vi "TDK正向工况电流-继电器控制 - 副本.vi"() -> ()   [LabVIEW 2020]
uses:
  <vilib>/Utility/file.llb/Read Delimited Spreadsheet (DBL).vi
  <instrlib>/TDK-Lambda G Series/TDK-Lambda G Series.lvlib
panel:
  out "耐久2":dbl[][](array[numeric])
  out "快充2":dbl[][](array[numeric])
  in  "耐久2":path
  in  "快充2":path
  in  "耐久循环次数2":i32
  in  "快充循环次数2":i32
  out "完成耐久循环 2":i32
  out "完成快充循环 2":i32
  in  "精度":i16
  out "?":bool
  in  "电源台数":dbl=3.0
  in  "TDK地址":refnum<visa-resource-name>="COM15"
  in  "耐久循环次数":i32
  in  "file path (dialog if empty) 2":path caption="耐久工况"
  out "耐久工况":string[][](table)
  out "快充工况":string[][](table)
  in  "file path (dialog if empty)":path caption="快充工况"
  out "已成大循环数":i32
  out "完成耐久循环":i32
  out "完成快充循环":i32
  in  "工况切换地址":refnum<visa-resource-name>
  in  "停止":bool
  in  "快充循环次数":i32
  in  "大循环次数":i32
  in  "耐久工况":cluster{"CH1":bool, "CH2":bool}
  in  "快充工况":cluster{"CH1":bool, "CH2":bool}
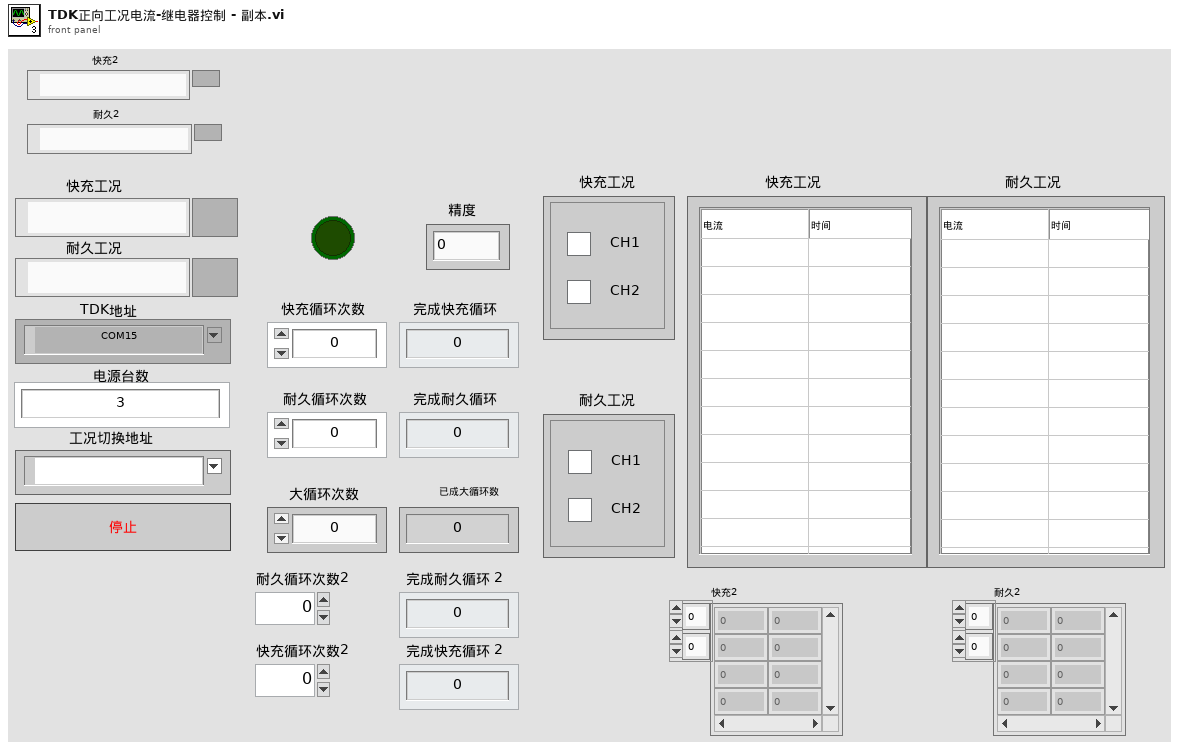
[diagram p1: front panel]
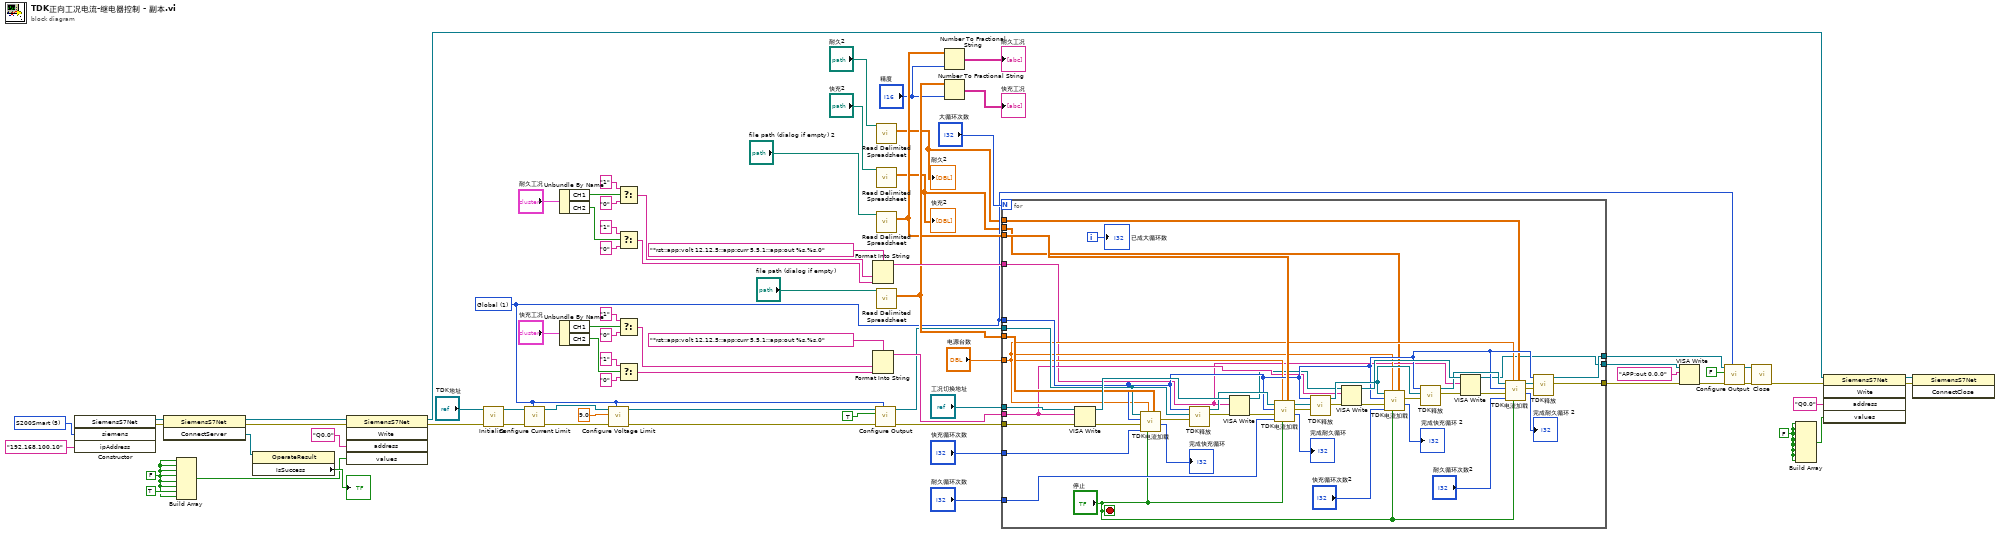
[diagram p0: block diagram]
diagram:
  w7 = FALSE ("元素")
  w18 = FALSE ("元素")
  w20 = 5 items=["S1200"=1, "S300"=2, "S400"=3, "S1500"=4, "S200Smart"=5, "S200"=6] ("siemens")
  w16 = u16 1 items=["Single", "Global"] ("Globalize (0: Single)")
  n1 = constructor class="SiemensS7Net"("siemens"=w20, "ipAddress"="192.168.100.10") -> (reference out=w27:refnum<k24>, error out=w28:errorcluster)  [unwired: 3 in, 3 out]
  n2 = invoke class="SiemensS7Net" method="ConnectServer"(reference=w27, error in=w28) -> (reference out=w23:refnum<k24>, error out=w22:errorcluster, "ConnectServer"=w25:refnum<k24>)  [unwired: 1 in]
  n3 = Build Array(w18, w18, w18, w18, w18, w18, TRUE ("元素"), w18) -> (w21:bool[])
  n4 = property class="OperateResult"(reference=w25) -> ("IsSuccess"=→"?":bool)  [unwired: 1 in, 2 out]
  n5 = invoke class="SiemensS7Net" method="Write"(reference=w23, error in=w22, "address"="Q0.0", "values"=w21) -> (reference out=w11:refnum<k24>, error out=w17:errorcluster)  [unwired: 1 in, 3 out]
  n6 = call <instrlib>:"Initialize.vi"("error in (no error)"=w17, "VISA resource name"="TDK地址") -> ("error out"=w41:errorcluster, "VISA resource name out"=w42:refnum<visa-resource-name>)  [unwired: 8 in]
  n7 = call <instrlib>:"Configure Current Limit.vi"("Globalize (0: Single)"=w16, "error in (no error)"=w41, "VISA resource name"=w42) -> ("error out"=w40:errorcluster, "VISA resource name out"=w39:refnum<visa-resource-name>)  [unwired: 7 in]
  n8 = Unbundle By Name("耐久工况") -> ("CH1"=w67:bool, "CH2"=w45:bool)
  n9 = Unbundle By Name("快充工况") -> ("CH1"=w77:bool, "CH2"=w46:bool)
  n10 = call <instrlib>:"Configure Voltage Limit.vi"("Globalize (0: Single)"=w16, "error in (no error)"=w40, "Voltage Limit (0V)"=9.0 ("Voltage Level (0.0 V)"), "VISA resource name"=w39) -> ("error out"=w37:errorcluster, "VISA resource name out"=w38:refnum<visa-resource-name>)  [unwired: 6 in]
  n11 = Select(t="1", s=w67, f="0") -> (s? t:f=w66:string)
  n12 = Select(t="1", s=w45, f="0") -> (s? t:f=w65:string)
  n13 = Select(t="1", s=w77, f="0") -> (s? t:f=w76:string)
  n14 = Select(t="1", s=w46, f="0") -> (s? t:f=w75:string)
  n15 = Format Into String(format string="*rst;:app:volt 12,12,5;:app:curr 5,5,1;:app:out %s,%s,0" ("格式字符串"), w66, w65) -> (resulting string=w59:string)  [unwired: 2 in, 1 out]
  n16 = Format Into String(format string="*rst;:app:volt 12,12,5;:app:curr 5,5,1;:app:out %s,%s,0" ("格式字符串"), w76, w75) -> (resulting string=w69:string)  [unwired: 2 in, 1 out]
  n17 = call <instrlib>:"Configure Output.vi"("Globalize (0: Single)"=w16, "error in (no error)"=w37, "Enable Output (False)"=TRUE, "VISA resource name"=w38) -> ("error out"=w35:errorcluster, "VISA resource name out"=w34:refnum<visa-resource-name>)  [unwired: 6 in]
  n18 = call-poly <vilib>:"Read Delimited Spreadsheet.vi"("file path (dialog if empty)"="耐久2") -> ("all rows"=w3:dbl[][])  [unwired: 9 in, 5 out]
  "耐久2" <- w3
  n19 = call-poly <vilib>:"Read Delimited Spreadsheet.vi"("file path (dialog if empty)"="快充2") -> ("all rows"=w4:dbl[][])  [unwired: 9 in, 5 out]
  "快充2" <- w4
  n20 = call-poly <vilib>:"Read Delimited Spreadsheet.vi"("file path (dialog if empty)"="file path (dialog if empty) 2") -> ("all rows"=w50:dbl[][])  [unwired: 9 in, 5 out]
  n21 = call-poly <vilib>:"Read Delimited Spreadsheet.vi"("file path (dialog if empty)"="file path (dialog if empty)") -> ("all rows"=w52:dbl[][])  [unwired: 9 in, 5 out]
  n22 = Number To Fractional String(number=w50, precision (6)="精度") -> (F-format string=→"耐久工况":string[][])  [unwired: 2 in]
  n23 = Number To Fractional String(number=w52, precision (6)="精度") -> (F-format string=→"快充工况":string[][])  [unwired: 2 in]
  n24 = for {
    N: "大循环次数" -> [_]
    tunnel: w69 -> [w87]
    tunnel: "工况切换地址" -> [w121]
    tunnel: w59 -> [w86]
    tunnel: [w79] -> w58
    tunnel: w34 -> [w104]
    tunnel: w52 -> [w119]
    tunnel: w50 -> [w116]
    tunnel: w35 -> [w115]
    tunnel: [w92] -> w14
    tunnel: "快充循环次数" -> [w106]
    tunnel: "耐久循环次数" -> [w105]
    tunnel: [w90] -> w15
    tunnel: w16 -> [w89]
    tunnel: "电源台数" -> [w88]
    tunnel: w3 -> [w82]
    tunnel: w4 -> [w81]
    i -> [w107]
    stop <- "停止" stop-if-true
    n25 = VISA Write(VISA resource name=w121, write buffer=w87, error in (no error)=w115) -> (VISA resource name out=w120:refnum<visa-resource-name>, error out=w114:errorcluster)  [unwired: 1 out]
    n26 = call "TDK电流加载.vi"("all rows"=w119, "停止"="停止", "电源台数"=w88, "循环次数"=w106, "error out"=w114, "Globalize (0: Single)"=w89, "VISA resource name out"=w104) -> ("已完成循环次数"=→"完成快充循环":i32, "error out 2"=w113:errorcluster)  [unwired: 2 in, 1 out]
    n27 = call "TDK释放.vi"("error out"=w113, "VISA resource name out"=w104, "Globalize (0: Single)"=w89) -> ("error out 2"=w112:errorcluster, "VISA resource name out 2"=w118:refnum<visa-resource-name>)  [unwired: 7 in]
    n28 = VISA Write(VISA resource name=w120, write buffer=w86, error in (no error)=w112) -> (VISA resource name out=w80:refnum<visa-resource-name>, error out=w111:errorcluster)  [unwired: 1 out]
    n29 = call "TDK电流加载.vi"("all rows"=w116, "停止"="停止", "电源台数"=w88, "循环次数"=w105, "error out"=w111, "Globalize (0: Single)"=w89, "VISA resource name out"=w118) -> ("已完成循环次数"=→"完成耐久循环":i32, "error out 2"=w110:errorcluster, "VISA resource name out 2"=w117:refnum<visa-resource-name>)  [unwired: 2 in]
    n30 = call "TDK释放.vi"("error out"=w110, "VISA resource name out"=w117, "Globalize (0: Single)"=w89) -> ("error out 2"=w93:errorcluster, "VISA resource name out 2"=w91:refnum<visa-resource-name>)  [unwired: 7 in]
    n31 = VISA Write(VISA resource name=w80, write buffer=w87, error in (no error)=w93) -> (VISA resource name out=w103:refnum<visa-resource-name>, error out=w100:errorcluster)  [unwired: 1 out]
    n32 = call "TDK电流加载.vi"("all rows"=w81, "停止"="停止", "电源台数"=w88, "循环次数"="快充循环次数2", "error out"=w100, "Globalize (0: Single)"=w89, "VISA resource name out"=w91) -> ("已完成循环次数"=→"完成快充循环 2":i32, "error out 2"=w99:errorcluster)  [unwired: 2 in, 1 out]
    n33 = call "TDK释放.vi"("error out"=w99, "VISA resource name out"=w91, "Globalize (0: Single)"=w89) -> ("error out 2"=w98:errorcluster, "VISA resource name out 2"=w102:refnum<visa-resource-name>)  [unwired: 7 in]
    n34 = VISA Write(VISA resource name=w103, write buffer=w86, error in (no error)=w98) -> (VISA resource name out=w79:refnum<visa-resource-name>, error out=w97:errorcluster)  [unwired: 1 out]
    n35 = call "TDK电流加载.vi"("all rows"=w82, "停止"="停止", "电源台数"=w88, "循环次数"="耐久循环次数2", "error out"=w97, "Globalize (0: Single)"=w89, "VISA resource name out"=w102) -> ("已完成循环次数"=→"完成耐久循环 2":i32, "error out 2"=w96:errorcluster, "VISA resource name out 2"=w101:refnum<visa-resource-name>)  [unwired: 2 in]
    n36 = call "TDK释放.vi"("error out"=w96, "VISA resource name out"=w101, "Globalize (0: Single)"=w89) -> ("error out 2"=w92:errorcluster, "VISA resource name out 2"=w90:refnum<visa-resource-name>)  [unwired: 7 in]
    "已成大循环数" <- w107
  }
  n37 = VISA Write(VISA resource name=w58, write buffer="APP:out 0,0,0" ("写入缓冲区"), error in (no error)=w14) -> (error out=w29:errorcluster)  [unwired: 2 out]
  n38 = call <instrlib>:"Configure Output.vi"("Globalize (0: Single)"=w16, "error in (no error)"=w29, "Enable Output (False)"=FALSE, "VISA resource name"=w15) -> ("error out"=w31:errorcluster, "VISA resource name out"=w32:refnum<visa-resource-name>)  [unwired: 6 in]
  n39 = call <instrlib>:"Close.vi"("error in (no error)"=w31, "VISA resource name"=w32) -> ("error out"=w9:errorcluster)  [unwired: 9 in]
  n40 = Build Array(w7, w7, w7, w7, w7, w7, w7, w7) -> (w12:bool[])
  n41 = invoke class="SiemensS7Net" method="Write"(reference=w11, error in=w9, "address"="Q0.0", "values"=w12) -> (reference out=w10:refnum<k24>, error out=w8:errorcluster)  [unwired: 1 in, 3 out]
  n42 = invoke class="SiemensS7Net" method="ConnectClose"(reference=w10, error in=w8) -> ()  [unwired: 1 in, 3 out]
